vi "Notify Subscribers.vi"(8 "error in (no error)":errorcluster, 10 "Topic Data":variant, 11 "Topic in":refnum<class "Topic.lvclass">) -> (0 "error out":errorcluster, 3 "Topic out":refnum<class "Topic.lvclass">)   [LabVIEW 2015, in "Mediator.lvlib" / "Topic.lvclass"]
uses:
  Topic.lvclass
  Transport/ITransport/ITransport.lvclass
  Topic.lvclass/Topic.ctl
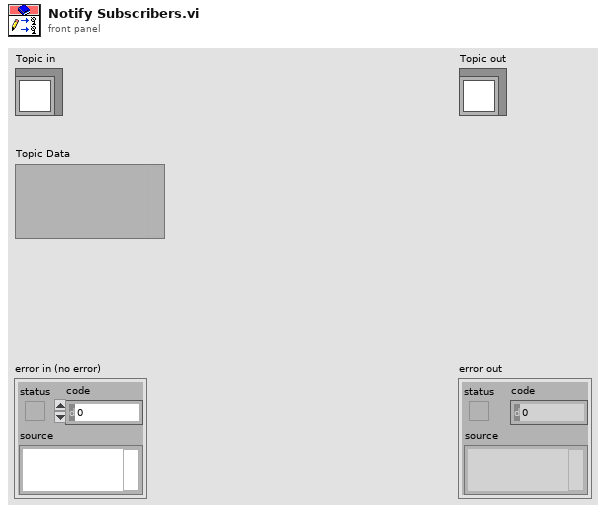
[diagram p1: front panel]
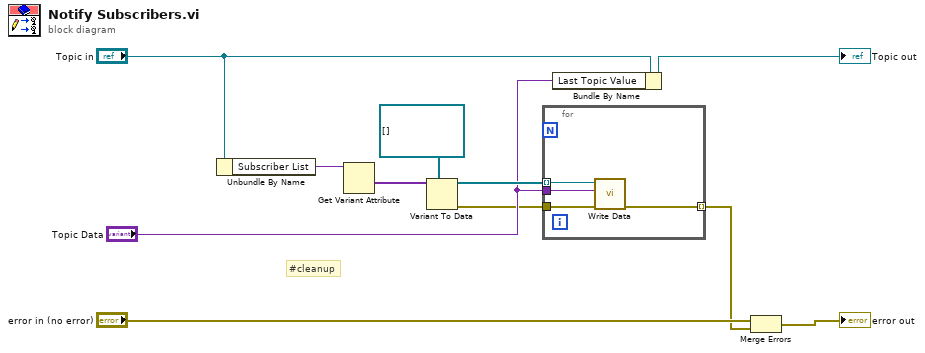
[diagram p0: block diagram]
diagram:
  # "#cleanup"
  n1 = Unbundle By Name("Topic in") -> ("Subscriber List"=w9:variant)
  n2 = Get Variant Attribute(Variant=w9) -> (values=w8:variant[])  [unwired: 3 in, 3 out]
  n3 = Variant To Data(type=refnum<class "ITransport.lvclass">[] [] ("Topic Enqueuer"), Variant=w8) -> (data=w5:refnum<class "ITransport.lvclass">[], error out=w2:errorcluster)  [unwired: 1 in]
  n4 = for {
    tunnel: w5 -> [w15] mode=indexing
    tunnel: "Topic Data" -> [w14]
    tunnel: w2 -> [w13]
    tunnel: [w12] -> w1 mode=indexing
    n5 = call-dynamic "Write Data.vi"("error in (no error)"=w13, "Anything"=w14, "ITransport in"=w15) -> ("error out"=w12:errorcluster)  [unwired: 7 in, 1 out]
  }
  n6 = Bundle By Name(cluster="Topic in", "Last Topic Value"="Topic Data") -> (→"Topic out":refnum<class "Topic.lvclass">)
  n7 = Merge Errors("error in (no error)", w1) -> (→"error out":errorcluster)
